vi "test.vi"() -> ()   [LabVIEW 2021]
uses:
  IChair/CushionModel.ctl
  ITable/TableclothType.ctl
  Chair/Chair.lvclass
  ChairWithTableAttached/ChairWithTableAttached.lvclass
  Table/Table.lvclass
  IChair/IChair.lvclass
  ITable/ITable.lvclass
panel:
  out "tablecloth results":string[](array[string])
  out "Cusioon  test Results":string[](array[string])
  out "Setup Result":string[](array[string])
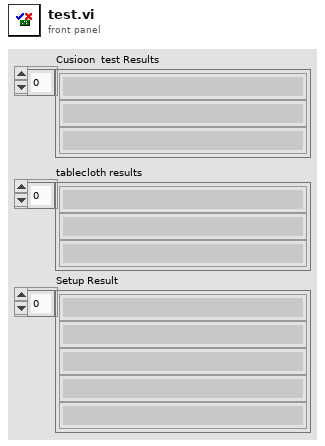
[diagram p1: front panel]
types:
  T1 = typedef "ITable.lvclass/TableclothType.ctl" = u16
  T2 = typedef "IChair.lvclass/CushionModel.ctl" = u16
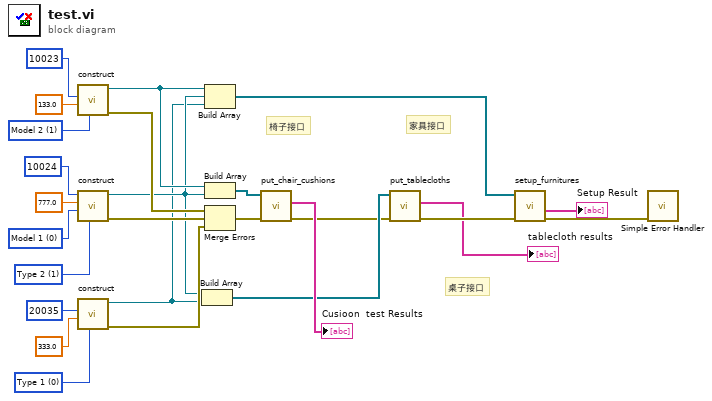
[diagram p0: block diagram]
diagram:
  w9 = T1 1 items=["Type 1", "Type 2"] ("tablecloth_type")
  w19 = T1 0 items=["Type 1", "Type 2"] ("tablecloth_type")
  w24 = T2 1 items=["Model 1", "Model 2"] ("cushion_model")
  w10 = T2 0 items=["Model 1", "Model 2"] ("cushion_model")
  # "家具接口"
  # "椅子接口"
  # "桌子接口"
  n1 = call "construct.vi"("cushion_model"=w24, "cost"=133.0 ("price"), "id"=u32 10023) -> ("error out"=w17:errorcluster, "Chair out"=w4:refnum<class "Chair.lvclass">)  [unwired: 7 in]
  n2 = call "construct.vi"("tablecloth_type"=w9, "cushion_model"=w10, "cost"=777.0 ("price"), "id"=u32 10024) -> ("error out"=w8:errorcluster, "ChairWithTableAttached out"=w3:refnum<class "ChairWithTableAttached.lvclass">)  [unwired: 6 in]
  n3 = call "construct.vi"("tablecloth_type"=w19, "cost"=333.0 ("price"), "id"=u32 20035) -> ("error out"=w16:errorcluster, "table out"=w2:refnum<class "Table.lvclass">)  [unwired: 7 in]
  n4 = Build Array(w3, w2) -> (w7:refnum<class "ITable.lvclass">[])
  n5 = Build Array(w4, w3, w2) -> (w23:refnum<class "IFurniture.lvclass">[])
  n6 = Build Array(w4, w3) -> (w18:refnum<class "IChair.lvclass">[])
  n7 = Merge Errors(w17, w8, w16) -> (w15:errorcluster)
  n8 = call "put_chair_cushions.vi"("error in"=w15, "chairs in"=w18) -> ("error out"=w6:errorcluster, "cushion results"=→"Cusioon  test Results":string[])  [unwired: 7 in, 1 out]
  n9 = call "put_tablecloths.vi"("error in (no error)"=w6, "tables in"=w7) -> ("error out"=w5:errorcluster, "tablecloth results"=→"tablecloth results":string[])  [unwired: 7 in, 1 out]
  n10 = call "setup_furnitures.vi"("error in"=w5, "furntures in"=w23) -> ("error out"=w13:errorcluster, "setup results"=→"Setup Result":string[])  [unwired: 7 in, 1 out]
  n11 = call <vilib>:"Simple Error Handler.vi"("error in (no error)"=w13) -> ()  [unwired: 4 in, 5 out]
